vi "Thev-Compute Px.vi"(0 "Ps":cdb[](array[numeric]), 5 "Zs":cdb[](array[numeric]), 7 "Zx":cdb[][](array[numeric])) -> (8 "Px":cdb[][](array[numeric]))   [LabVIEW 2015]
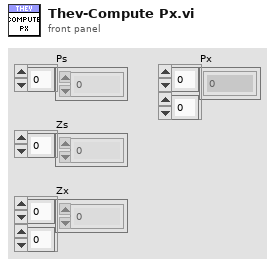
[diagram p1: front panel]
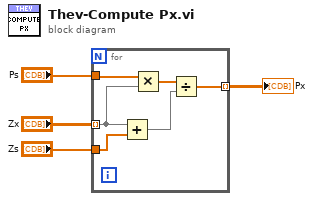
[diagram p0: block diagram]
diagram:
  n1 = for {
    tunnel: "Zx" -> [w8] mode=indexing
    tunnel: "Ps" -> [w10]
    tunnel: "Zs" -> [w7]
    tunnel: [w5] -> w1 mode=indexing
    n2 = Add(x=w8, y=w7) -> (x+y=w6:cdb[])
    n3 = Multiply(x=w10, y=w8) -> (x*y=w9:cdb[])
    n4 = Divide(x=w9, y=w6) -> (x/y=w5:cdb[])
  }
  "Px" <- w1
